vi "Test - Navigator Target.vi"() -> ()   [LabVIEW 2019]
doc: "This VI serves as the target for a scripting VI. Do not save changes to this VI."
panel:
  in  "message":string
  # "Select Help>>Show Context Help and move the cursor over the VI icon to display help for this VI.\n\nDO NOT SAVE CHANGES TO THIS VI. This VI serves as the target for a scripting VI. Therefore, changing this VI might prevent the scripting VIs from demonstrating its scripting task."
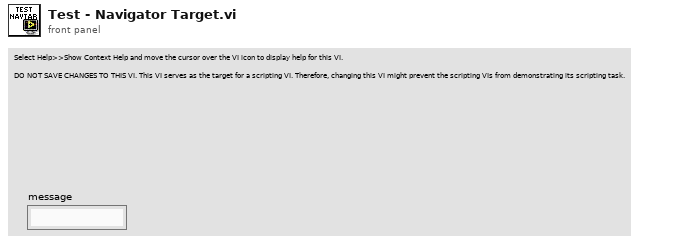
[diagram p1: front panel]
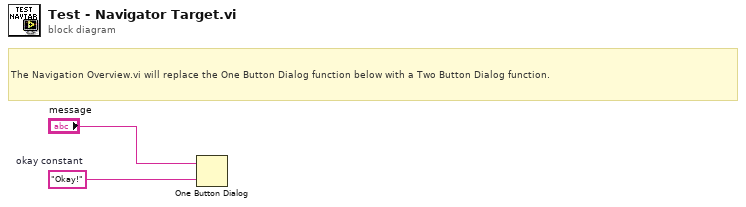
[diagram p0: block diagram]
diagram:
  w1 = "Okay!"  # okay constant
  # "The Navigation Overview.vi will replace the One Button Dialog function below with a Two Button Dialog function."
  n1 = One Button Dialog(message="message", button name ("OK")=w1) -> ()  [unwired: 1 out]
